vi "Tusk.ValidateTusk (Local).vi"(8 "error in (no error)":errorcluster, 11 "Tusk in":refnum<class "Tusk.lvclass">) -> (0 "error out":errorcluster, 2 "Valid?":bool, 3 "Tusk out":refnum<class "Tusk.lvclass">)   [LabVIEW 2018, in "Application.lvlib" / "Tusk.lvclass"]
uses:
  Tusk.lvclass
  Tusk.lvclass/Tusk.ctl
  Dictionary Class/Dictionary.lvclass/Dictionary.ctl
  Exceptions Class/VIs/Invalid Name Format.vi
  Dictionary Class/VIs/Get Data DVR.vi
  Dictionary Class/Dictionary.lvclass
  Exceptions Class/Exceptions.lvclass
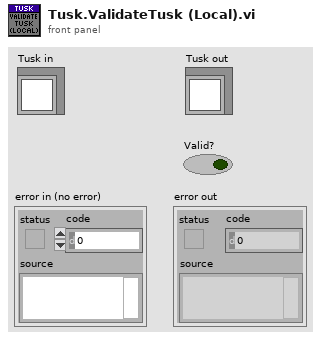
[diagram p1: front panel]
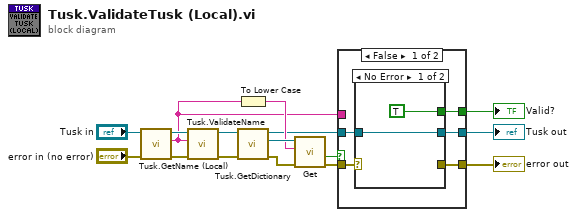
[diagram p0: block diagram]
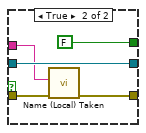
[diagram p3: hidden frame]
diagram:
  n1 = call "Tusk.GetName (Local).vi"("error in (no error)"="error in (no error)", "Tusk in"="Tusk in") -> ("error out"=w3:errorcluster, "Name(Local)"=w1:string, "Tusk out"=w2:refnum<class "Tusk.lvclass">)  [unwired: 7 in]
  n2 = call "Tusk.ValidateName.vi"("error in (no error)"=w3, "Name"=w1, "Tusk in"=w2) -> ("error out"=w13:errorcluster, "Tusk out"=w14:refnum<class "Tusk.lvclass">)  [unwired: 7 in]
  n3 = To Lower Case(string=w1) -> (all lower case string=w12:string)
  n4 = call "Tusk.GetDictionary.vi"("error in (no error)"=w13, "Tusk in"=w14) -> ("error out"=w16:errorcluster, "Dictionary"=w15:refnum<class "Dictionary.lvclass">, "Tusk out"=w11:refnum<class "Tusk.lvclass">)  [unwired: 7 in]
  n5 = call "Get.vi"("error in (no error)"=w16, "Key"=w12, "Dictionary in"=w15) -> ("error out"=w10:errorcluster, "Success?"=w9:bool)  [unwired: 5 in, 2 out]
  n6 = case shown="False" w9 {
    tunnel: w11 -> [w18 w29]
    tunnel: w10 -> [w20 w30]
    tunnel: [w17 w29] -> w6
    tunnel: [w19 w28] -> w8
    tunnel: w1 -> [_ w27]
    tunnel: [w21 FALSE] -> w7
    frame False {
      n7 = case shown="No Error" w20 {
        selector: w20 -> [_ w25]
        tunnel: [TRUE _] -> w21
        tunnel: [_ w25] -> w19
        tunnel: w18 -> [w22 w24]
        tunnel: [w22 w24] -> w17
        frame No Error {
        }
        frame Error {
        }
      }
    }
    frame True {
      n8 = call "Name (Local) Taken.vi"("error in (no error)"=w30, "Name (Local)"=w27) -> ("error out"=w28:errorcluster)  [unwired: 9 in]
    }
  }
  "Tusk out" <- w6
  "error out" <- w8
  "Valid?" <- w7
